vi "Switch LED on-off.vi"(8 "error in":errorcluster, 9 "LED On/Off":bool, 10 "LED":enum8{"Red", "UV", "Green", "Blue"}(ring), 11 "LED handle in":refnum<visa-resource-name>) -> (0 "error out":errorcluster {"code" format="%.0x"}, 3 "LED handle out":refnum<visa-resource-name> caption="instrument handle out")   [LabVIEW 2017]
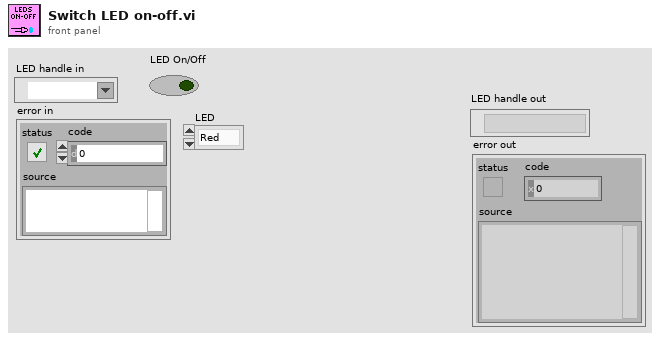
[diagram p1: front panel]
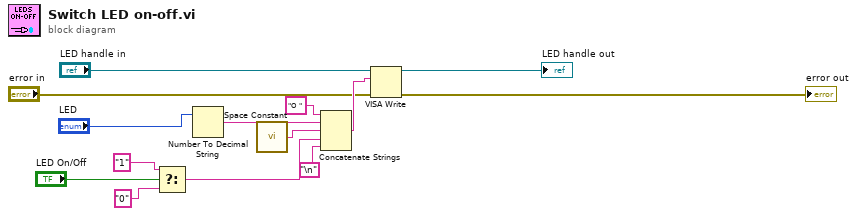
[diagram p0: block diagram]
diagram:
  n1 = Select(t="1", s="LED On/Off", f="0" ("String")) -> (s? t:f=w4:string)
  n2 = Number To Decimal String(number="LED") -> (decimal integer string=w6:string)  [unwired: 1 in]
  n3 = call <vilib>:"Space Constant.vi"() -> ("String"=w8:string)
  n4 = Concatenate Strings("O " ("string"), w6, w8, w4, "\n") -> (w14:string)
  n5 = VISA Write(VISA resource name="LED handle in", write buffer=w14, error in (no error)="error in") -> (VISA resource name out=→"LED handle out":refnum<visa-resource-name>, error out=→"error out":errorcluster)  [unwired: 1 out]
